vi "SetValueByArrayName.vi"(0 "VI Reference In":refnum<vi>, 2 "delimiter (>>)":string=">>", 5 "Control Path":string, 7 "Name Array":T1[](array[typedef]), 11 "Error In":errorcluster) -> (4 "VI Reference Out":refnum<vi>, 15 "Error Out":errorcluster)   [LabVIEW 2016, in "Drona.lvlib" / "ControlValue.lvlib" / "StimulusMCListbox.lvlib"]
doc: "Sets value(signaling) for the multi select multi column listbox control whose first column item names with its occurrence are specified. Set the value as 1 in occurrence to select the first occurrence of an item. \n\nThe input control name is given as a string , incase of path, use delimiters inbetween the path."
uses:
  StimulusMCListbox.lvlib
  typedef/Name&Occurrence.ctl
  <vilib>/Utility/error.llb/Error Cluster From Error Code.vi
  <vilib>/ErrorRing/Error Ring.xnode
  <userlib>/_OpenG.lib/array/array.llb/Search 1D Array (String)__ogtk.vi
  Drona.lvlib
  Get/GetControlRef/GetControlRef.lvlib
  ControlValue.lvlib
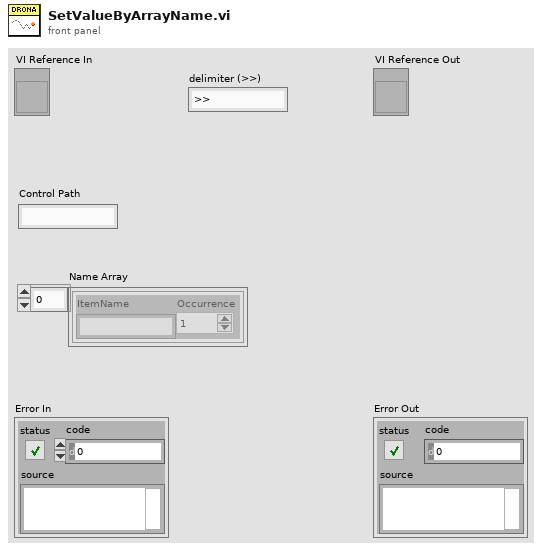
[diagram p1: front panel]
types:
  T1 = typedef "Drona.lvlib/ControlValue.lvlib/Name&Occurrence.ctl" = cluster{"ItemName":string, "Occurrence":i32}
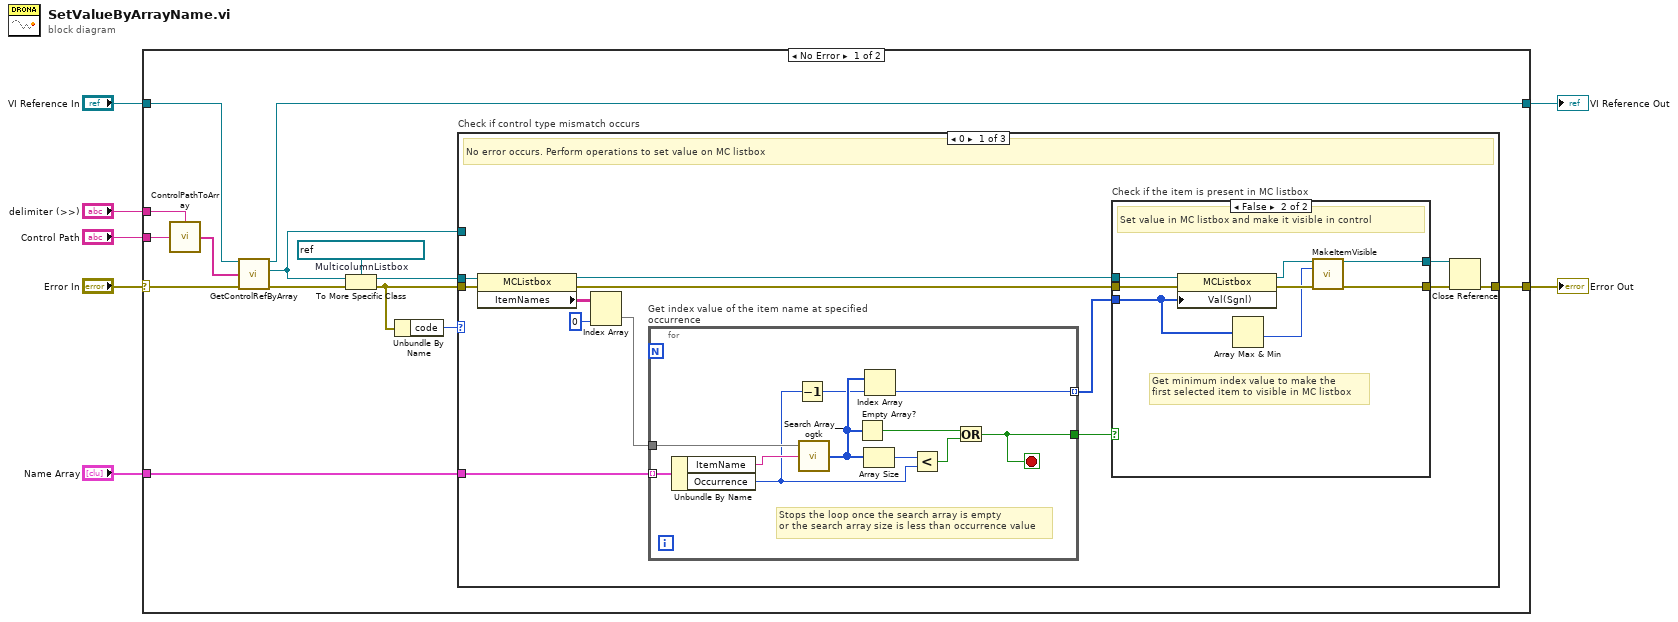
[diagram p0: block diagram]
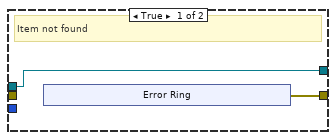
[diagram p2: hidden frame]
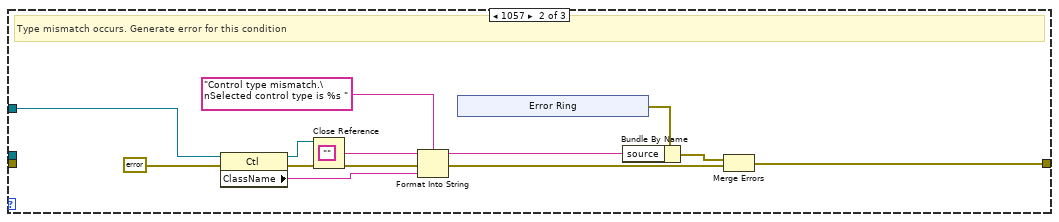
[diagram p3: hidden frame]
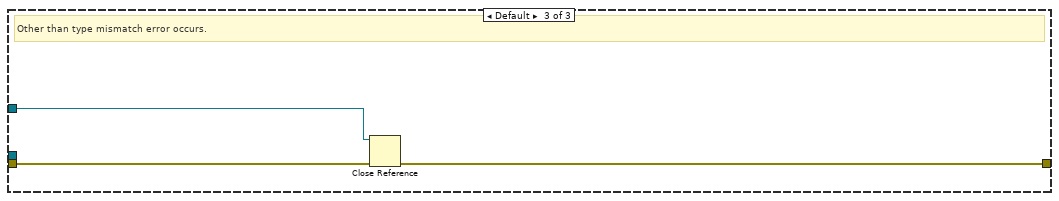
[diagram p4: hidden frame]
diagram:
  n1 = case shown="No Error" "Error In" {
    selector: "Error In" -> [w16 w83]
    tunnel: [w17 w83] -> w6
    tunnel: "VI Reference In" -> [w15 w82]
    tunnel: "Control Path" -> [w19 _]
    tunnel: [w12 w82] -> w3
    tunnel: "delimiter (>>)" -> [w18 _]
    tunnel: "Name Array" -> [w11 _]
    frame No Error {
      w21 = refnum<vi> refnum  # MulticolumnListbox
      n2 = call "ControlPathToArray.vi"("Control Name"=w19, "delimiter (>>)"=w18) -> ("Control Path"=w14:string[])
      n3 = call "GetControlRefByArray.vi"("VI Reference In"=w15, "Control Path"=w14, "error In"=w16) -> ("VI Reference Out"=w12:refnum<vi>, "Ctl Refnum"=w8:refnum<vi>, "error out"=w13:errorcluster)  [unwired: 10 in]
      n4 = To More Specific Class(target class=w21, reference=w8, error in=w13) -> (specific class reference=w20:refnum<vi>, error out=w10:errorcluster)
      n5 = Unbundle By Name(w10) -> ("code"=w9:i32)
      n6 = case "Check if control type mismatch occurs" shown="0" w9 {
        tunnel: w10 -> [w34 _ w81]
        tunnel: w20 -> [w33 _ _]
        tunnel: [w32 w61 w80] -> w17
        tunnel: w11 -> [w29 _ _]
        tunnel: w8 -> [_ w62 w79]
        frame 0 {
          # "No error occurs. Perform operations to set value on MC listbox"
          n7 = property class="MCListbox"(reference=w33, error in=w34) -> (reference out=w27:refnum<vi>, error out=w28:errorcluster, "ItemNames"=w24:string[][])
          n8 = Index Array(array=w24, index (col)=0 ("disabled index (col)")) -> (element=w22:string[])  [unwired: 1 in]
          n9 = for "Get index value of the item name at specified occurrence" {
            tunnel: w22 -> [w44]
            tunnel: w29 -> [w45] mode=indexing
            tunnel: [w36] -> w26 mode=indexing
            tunnel: [w35] -> w25
            stop <- w35 stop-if-true
            # "Stops the loop once the search array is empty \nor the search array size is less than occurrence value"
            n10 = Unbundle By Name(w45) -> ("ItemName"=w43:string, "Occurrence"=w38:i32)
            n11 = Decrement(x=w38) -> (x-1=w37:i32)
            n12 = call-poly <userlib>:"Search Array__ogtk.vi"("Array"=w44, "Element Data"=w43) -> ("Indices of Elements"=w39:i32[])  [unwired: 7 in]
            n13 = Empty Array?(array=w39) -> (empty?=w40:bool)
            n14 = Array Size(array=w39) -> (size(s)=w42:i32)
            n15 = Index Array(array=w39, index=w37) -> (element=w36:i32)
            n16 = Less?(x=w42, y=w38) -> (x < y?=w41:bool)
            n17 = Or(x=w40, y=w41) -> (x .or. y?=w35:bool)
          }
          n18 = case "Check if the item is present in MC listbox" shown="False" w25 {
            tunnel: [w47 w59] -> w31
            tunnel: [w46 w57] -> w30
            tunnel: w28 -> [_ w55]
            tunnel: w27 -> [w46 w54]
            tunnel: w26 -> [_ w53]
            frame True {
              # "Item not found"
              n19 = xnode "Error Ring"() -> ("error out"=w47:errorcluster)
            }
            frame False {
              # "Get minimum index value to make the \nfirst selected item to visible in MC listbox"
              # "Set value in MC listbox and make it visible in control"
              n20 = property class="MCListbox"(reference=w54, error in=w55, "Val(Sgnl)"=w53) -> (reference out=w58:refnum<vi>, error out=w60:errorcluster)
              n21 = Array Max & Min(array=w53) -> (min value=w56:i32)  [unwired: 3 out]
              n22 = call "MakeItemVisible.vi"("MC ListBox Ref In"=w58, "Item Index"=w56, "Error In"=w60) -> ("MC ListBox Ref Out"=w57:refnum<vi>, "Error Out"=w59:errorcluster)  [unwired: 11 in]
            }
          }
          n23 = Close Reference(reference=w30, error in (no error)=w31) -> (error out=w32:errorcluster)
        }
        frame 1057 {
          # "Type mismatch occurs. Generate error for this condition"
          n24 = property class="Ctl"(reference=w62, error in=errorcluster {"status"=FALSE, "code"=0, "source"=""} ("error out")) -> (reference out=w63:refnum<vi>, error out=w73:errorcluster, "ClassName"=w70:string)
          n25 = Close Reference(reference=w63, error in (no error)=w73) -> (error out=w64:errorcluster)
          n26 = Format Into String(format string="Control type mismatch.\nSelected control type is %s ", initial string="", error in=w64, w70) -> (resulting string=w67:string, error out=w65:errorcluster)
          n27 = xnode "Error Ring"() -> ("error out"=w68:errorcluster)
          n28 = Bundle By Name(cluster=w68, "source"=w67) -> (w66:errorcluster)
          n29 = Merge Errors(w66, w65) -> (w61:errorcluster)
        }
        frame Default {
          # "Other than type mismatch error occurs."
          n30 = Close Reference(reference=w79, error in (no error)=w81) -> (error out=w80:errorcluster)
        }
      }
    }
    frame Error {
    }
  }
  "Error Out" <- w6
  "VI Reference Out" <- w3
